vi "gyro -- launch async sourcer.vi"(11 "sourcer pair":T1) -> (2 "reference out":refnum<vi>, 3 "fitter pair OUT":T1)   [LabVIEW 2018]
uses:
  server talkback message type.ctl
  server talkto message type.ctl
  server talk-to-back pair.ctl
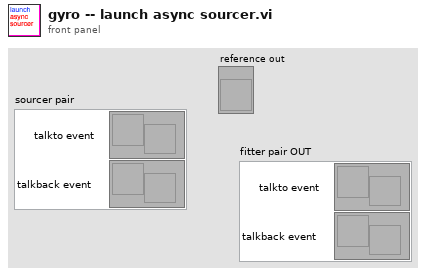
[diagram p1: front panel]
types:
  T1 = typedef "server talk-to-back pair.ctl" = cluster{"talkback event":refnum<user-event>, "talkto event":refnum<user-event>}
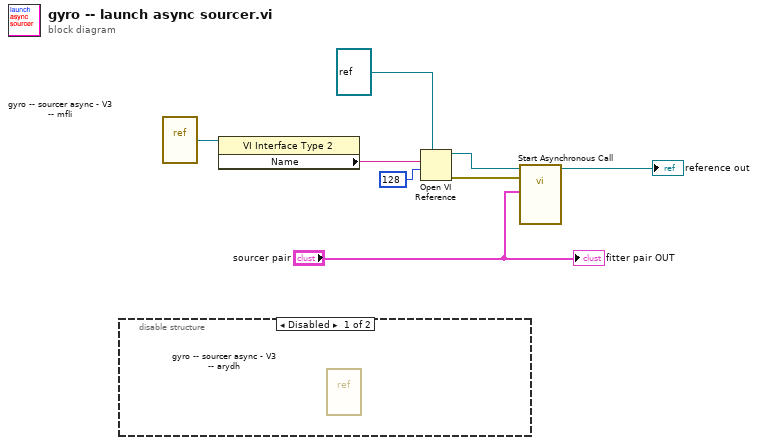
[diagram p0: block diagram]
diagram:
  n1 = disable-structure shown="Disabled" {
    frame Disabled {
      n2 = vi-ref "gyro -- sourcer async - V3 -- arydh.vi"() -> ()  [unwired: 1 out]
    }
    frame Enabled {
    }
  }
  n3 = vi-ref "gyro -- sourcer async - V3 -- mfli.vi"() -> (w7:refnum<vi>)
  n4 = property class="VI Interface Type 2"(reference=w7) -> ("Name"=w6:string)  [unwired: 1 in, 2 out]
  n5 = Open VI Reference(type specifier VI Refnum (for type only)=refnum<vi> refnum, vi path=w6, options=128) -> (vi reference=w3:refnum<vi>, error out=w2:errorcluster)  [unwired: 3 in]
  n6 = call-by-ref "Start Asynchronous Call"(reference=w3, error in=w2, "pll event pair"="sourcer pair") -> (reference out=→"reference out":refnum<vi>)  [unwired: 11 in, 1 out]
  "fitter pair OUT" <- "sourcer pair"
